vi "UDP-Create.vi"(9 "Ethernet II Params":T1 {"Destination MAC" format="%.0x"; "Source MAC" format="%.02x"; "EtherType" format="%.0x"}, 10 "IPv4 Params":T2, 11 "UDP Params":T3) -> (1 "Ethernet Frame\nU64":u64[](array[numeric]) format="%016x", 2 "Ethernet Frame\nsize":i32, 3 "Ethernet Frame":u8[](array[numeric])=[0, 224, 247, 38, 63, 233, 8, 0, 32, 134, 53, 75, 8, 0, 69, 0, 0, 40, 171, 75, 64, 0, 255, 17, 246, 252, 139, 133, 217, 110, 139, 133, 233, 2, 153, 208, 4, 63, 0, 20, 0, 0, 114, 40, 104, 101, 108, 108, 111, 104, 101, 108, 108, 111] format="%.0x")   [LabVIEW 2018]
panel:
  out "Array":u8[][](array[numeric]) format="%.0x"
  out "Raw \nUDP Size":i32=20 format="%.0x"
  out "String":string="static u8 var[] = {\r\n0x00, 0xE0, 0xF7, 0x26, 0x3F, 0xE9, 0x08, 0x00, \r\n0x20, 0x86, 0x35, 0x4B, 0x08, 0x00, 0x45, 0x00, \r\n0x00, 0x28, 0xAB, 0x4B, 0x40, 0x00, 0xFF, 0x11, \r\n0xF6, 0xFC, 0x8B, 0x85, 0xD9, 0x6E, 0x8B, 0x85, \r\n0xE9, 0x02, 0x99, 0xD0, 0x04, 0x3F, 0x00, 0x14, \r\n0x00, 0x00, 0x72, 0x28, 0x68, 0x65, 0x6C, 0x6C};"
  out "Raw UDP":u8[](array[numeric])=[153, 208, 4, 63, 0, 20, 0, 0, 114, 40, 104, 101, 108, 108, 111, 104, 101, 108, 108, 111] format="%.0x"
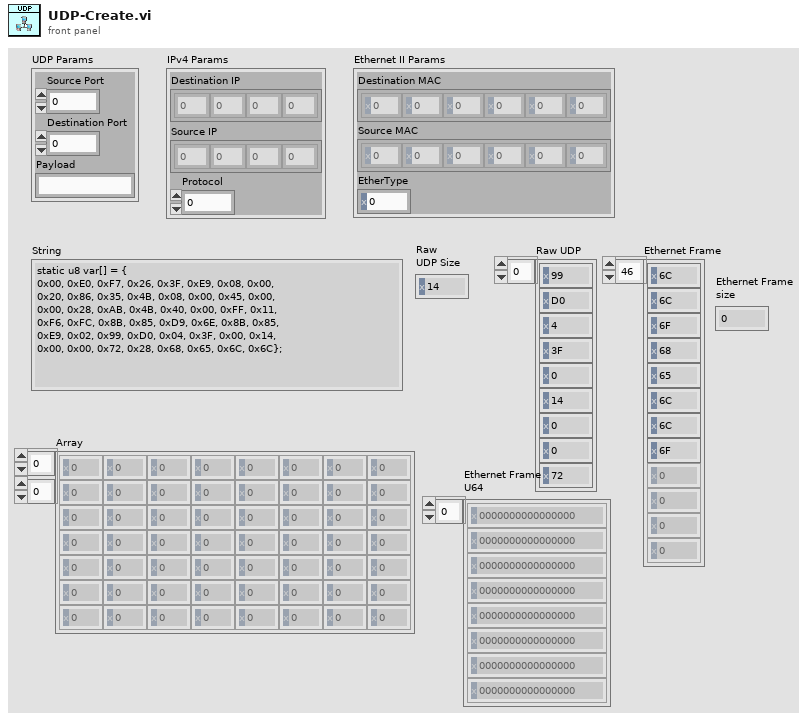
[diagram p1: front panel]
types:
  T1 = cluster{"Destination MAC":u8[], "Source MAC":u8[], "EtherType":u16}
  T2 = cluster{"Destination IP":u8[], "Source IP":u8[], "Protocol":u8}
  T3 = cluster{"Source Port":u16, "Destination Port":u16, "Payload":string}
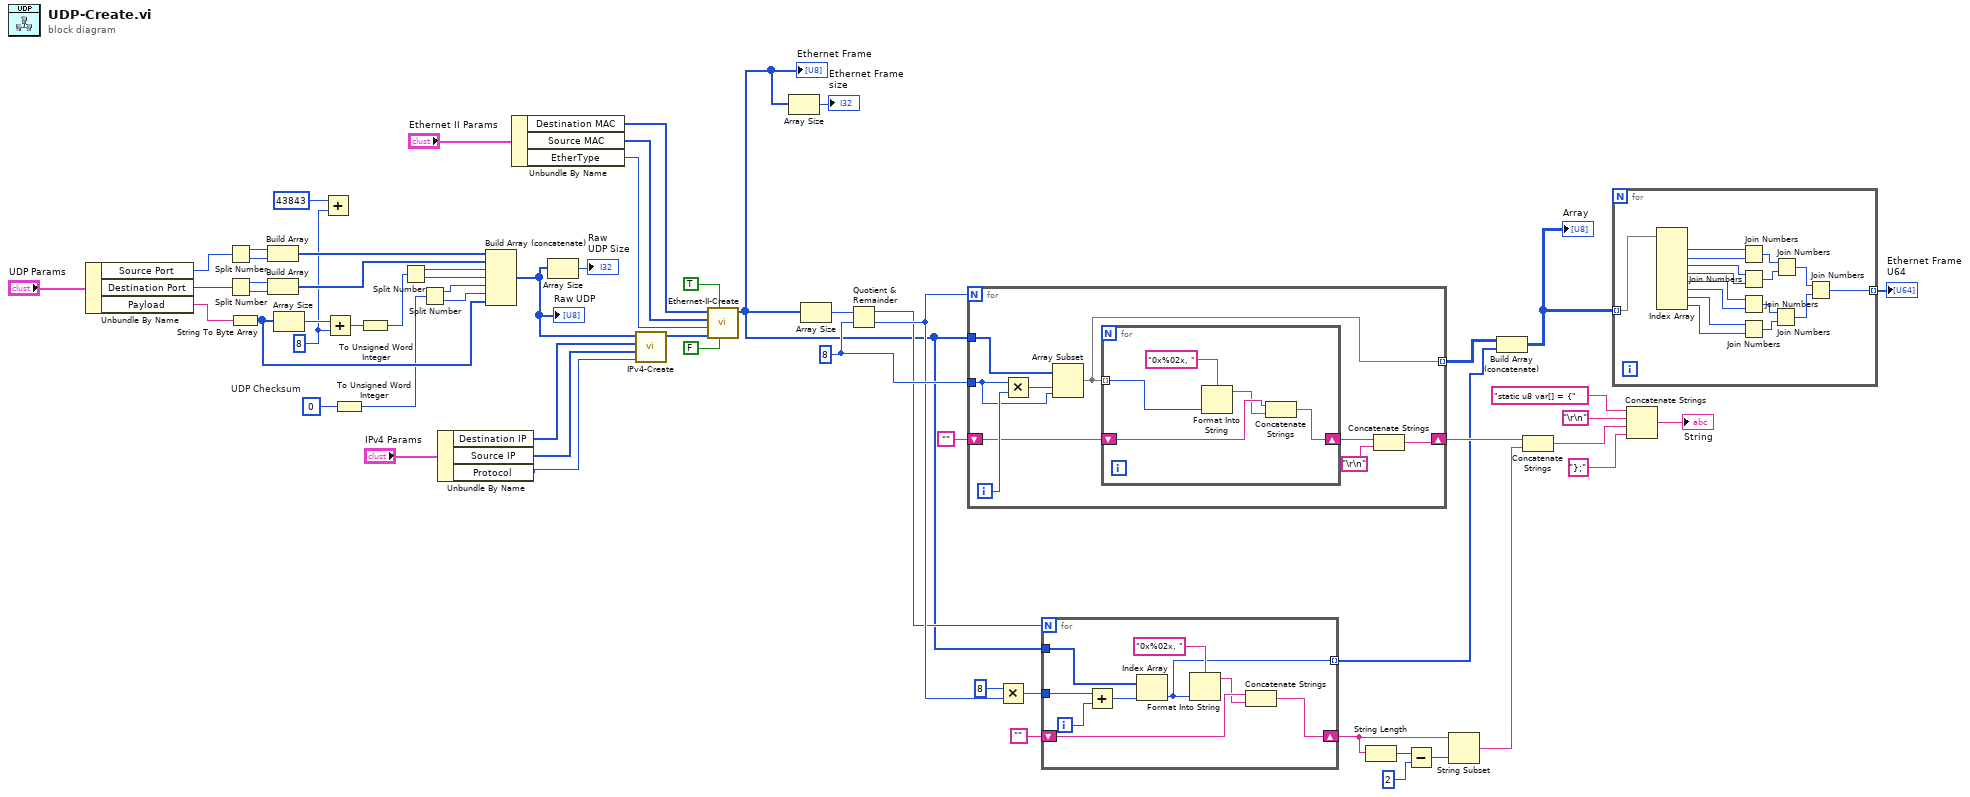
[diagram p0: block diagram]
diagram:
  w36 = u16 0  # UDP Checksum
  w45 = 8 ("y")
  w47 = u16 8 ("y")
  n1 = Unbundle By Name("UDP Params") -> ("Source Port"=w17:u16, "Destination Port"=w16:u16, "Payload"=w15:string)
  n2 = Split Number(x=w17) -> (hi(x)=w59:u8, lo(x)=w60:u8)
  n3 = Split Number(x=w16) -> (hi(x)=w57:u8, lo(x)=w58:u8)
  n4 = String To Byte Array(string=w15) -> (unsigned byte array=w40:u8[])
  n5 = Build Array(w59, w60) -> (w56:u8[])
  n6 = Build Array(w57, w58) -> (w55:u8[])
  n7 = Array Size(array=w40) -> (size(s)=w54:i32)
  n8 = Add(x=u16 43843, y=w47) -> ()  [unwired: 1 out]
  n9 = Add(x=w54, y=w47) -> (x+y=w53:i32)
  n10 = To Unsigned Word Integer(number=w36) -> (unsigned 16bit integer=w37:u16)
  n11 = To Unsigned Word Integer(number=w53) -> (unsigned 16bit integer=w50:u16)
  n12 = Split Number(x=w50) -> (hi(x)=w52:u8, lo(x)=w51:u8)
  n13 = Split Number(x=w37) -> (hi(x)=w39:u8, lo(x)=w38:u8)
  n14 = Unbundle By Name("IPv4 Params") -> ("Destination IP"=w13:u8[], "Source IP"=w12:u8[], "Protocol"=w11:u8)
  n15 = Build Array (concatenate)(w56, w55, w52, w51, w39, w38, w40) -> (w35:u8[])
  "Raw UDP" <- w35
  n16 = Unbundle By Name("Ethernet II Params") -> ("Destination MAC"=w7:u8[], "Source MAC"=w8:u8[], "EtherType"=w9:u16)
  n17 = Array Size(array=w35) -> (size(s)=→"Raw \nUDP Size":i32)
  n18 = call "IPv4-Create.vi"("Protocol"=w11, "Source IP"=w12, "Destination IP"=w13, "IPv4\nPayload"=w35) -> ("IPv4 Packet"=w49:u8[])  [unwired: 7 in]
  n19 = call "Ethernet-II-Create.vi"("Add CRC32?"=FALSE, "PadLen?"=TRUE, "Payload (in)"=w49, "EtherType"=w9, "Source MAC"=w8, "Destination MAC"=w7) -> ("Ethernet Frame (out)"=w20:u8[])  [unwired: 5 in]
  "Ethernet Frame" <- w20
  n20 = Array Size(array=w20) -> (size(s)=→"Ethernet Frame\nsize":i32)
  n21 = Array Size(array=w20) -> (size(s)=w46:i32)
  n22 = Quotient & Remainder(x=w46, y=w45) -> (x-y*floor(x/y)=w32:i32, floor(x/y)=w33:i32)
  n23 = for {
    N: w33 -> [_]
    tunnel: w45 -> [w67]
    shift-right: [w61] -> w23
    shift-left: "" -> [w66]
    tunnel: [w64] -> w6 mode=indexing
    tunnel: w20 -> [w65]
    i -> [w68]
    n24 = Multiply(x=w67, y=w68) -> (x*y=w69:i32)
    n25 = Array Subset(array=w65, index=w69, length=w67) -> (w64:u8[])
    n26 = for {
      tunnel: w64 -> [w73] mode=indexing
      shift-right: [w72] -> w63
      shift-left: w66 -> [w71]
      n27 = Format Into String(format string="0x%02x, ", w73) -> (resulting string=w70:string)  [unwired: 2 in, 1 out]
      n28 = Concatenate Strings(w71, w70) -> (w72:string)
    }
    n29 = Concatenate Strings(w63, "\r\n") -> (w61:string)
  }
  n30 = Multiply(x=8, y=w33) -> (x*y=w30:i32)
  n31 = for {
    N: w32 -> [_]
    tunnel: w30 -> [w81]
    shift-right: [w78] -> w25
    shift-left: "" -> [w80]
    tunnel: w20 -> [w79]
    tunnel: [w75] -> w5 mode=indexing
    i -> [w82]
    n32 = Add(x=w81, y=w82) -> (x+y=w83:i32)
    n33 = Index Array(array=w79, index=w83) -> (element=w75:u8)
    n34 = Format Into String(format string="0x%02x, ", w75) -> (resulting string=w76:string)  [unwired: 2 in, 1 out]
    n35 = Concatenate Strings(w80, w76) -> (w78:string)
  }
  n36 = String Length(string=w25) -> (length=w27:i32)
  n37 = Subtract(x=w27, y=2) -> (x-y=w28:i32)
  n38 = String Subset(string=w25, length (rest)=w28) -> (substring=w24:string)  [unwired: 1 in]
  n39 = Build Array (concatenate)(w6, w5) -> (w4:u8[][])
  "Array" <- w4
  n40 = Concatenate Strings(w23, w24) -> (w21:string)
  n41 = for {
    tunnel: w4 -> [w99] mode=indexing
    tunnel: [w84] -> w3 mode=indexing
    n42 = Index Array(array=w99) -> (element #1=w98:u8, element #2=w97:u8, element #3=w96:u8, element #4=w95:u8, element #5=w94:u8, element #6=w93:u8, element #7=w92:u8, element #8=w91:u8)  [unwired: 8 in]
    n43 = Join Numbers(hi=w98, lo=w97) -> ((hi.lo)=w90:u16)
    n44 = Join Numbers(hi=w96, lo=w95) -> ((hi.lo)=w89:u16)
    n45 = Join Numbers(hi=w94, lo=w93) -> ((hi.lo)=w88:u16)
    n46 = Join Numbers(hi=w92, lo=w91) -> ((hi.lo)=w87:u16)
    n47 = Join Numbers(hi=w88, lo=w87) -> ((hi.lo)=w86:u32)
    n48 = Join Numbers(hi=w90, lo=w89) -> ((hi.lo)=w85:u32)
    n49 = Join Numbers(hi=w85, lo=w86) -> ((hi.lo)=w84:u64)
  }
  "Ethernet Frame\nU64" <- w3
  n50 = Concatenate Strings("static u8 var[] = {" ("string"), "\r\n", w21, "};" ("string")) -> (→"String":string)
